vi "sub match keyword two value.vi"(8 "error in":errorcluster, 10 "keyword":string[](array[string]), 11 "string":string) -> (0 "error out":errorcluster, 2 "matched pairs (exist)":T1(array[cluster]), 3 "matched pairs (all)":T1(array[cluster]), 5 "remain string":string)   [LabVIEW 2018, in "Data Parser.lvclass"]
uses:
  Data Parser.lvclass
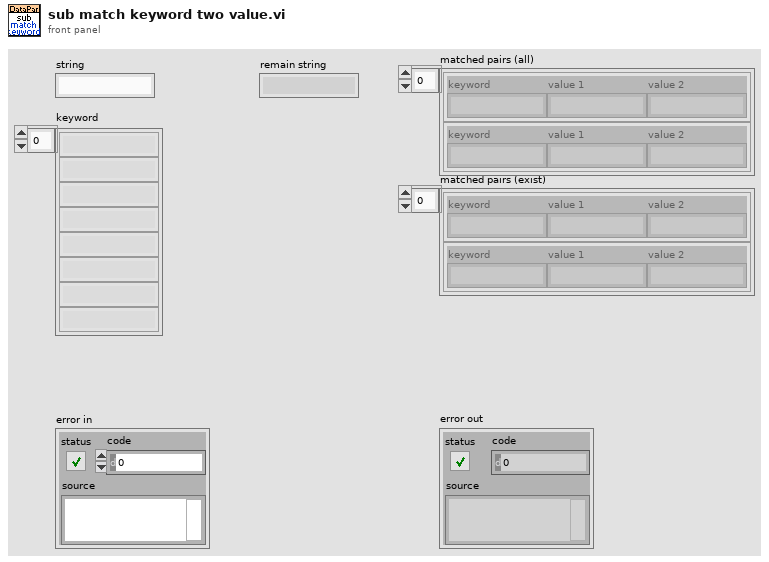
[diagram p1: front panel]
types:
  T1 = cluster{"keyword":string, "value 1":string, "value 2":string}[]
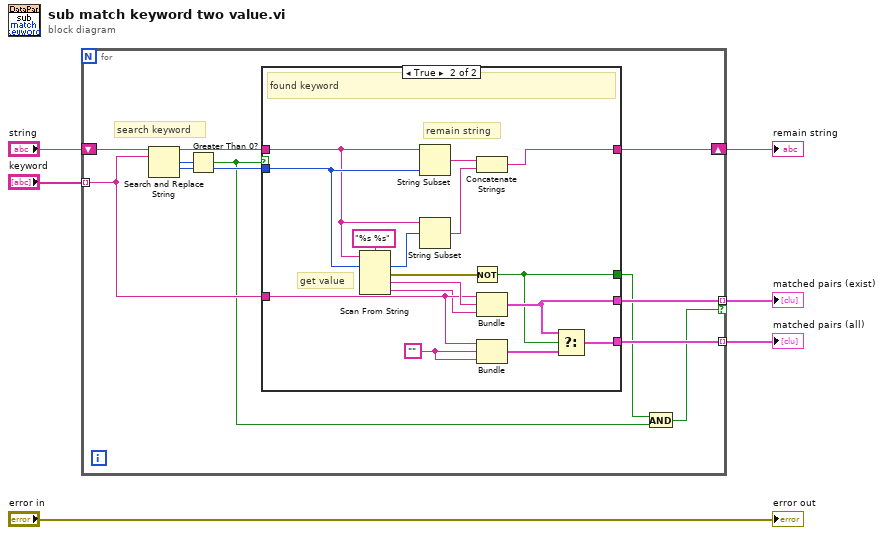
[diagram p0: block diagram]
diagram:
  n1 = for {
    tunnel: "keyword" -> [w12] mode=indexing
    shift-right: [w14] -> w3
    shift-left: "string" -> [w17]
    tunnel: [w13] -> w6 mode=indexing if=w7
    tunnel: [w11] -> w1 mode=indexing
    # "search keyword"
    n2 = Search and Replace String(input string=w17, search string=w12) -> (result string=w15:string, number of replacements=w10:i32, offset past replacement=w16:i32)  [unwired: 6 in, 1 out]
    n3 = Greater Than 0?(x=w10) -> (x > 0?=w9:bool)
    n4 = case shown="True" w9 {
      tunnel: w16 -> [_ w32]
      tunnel: w15 -> [w18 w31]
      tunnel: [w18 w27] -> w14
      tunnel: [_ w26] -> w13
      tunnel: w12 -> [_ w25]
      tunnel: [_ w23] -> w11
      tunnel: [_ w21] -> w8
      frame False {
        # "not found"
      }
      frame True {
        w20 = ""
        # "remain string"
        # "get value"
        # "found keyword"
        n5 = Scan From String(format string="%s %s", input string=w31, initial scan location=w32) -> (offset past scan=w30:u32, error out=w22:errorcluster, output 1=w33:string, output 2=w19:string)  [unwired: 3 in, 1 out]
        n6 = String Subset(string=w31, length (rest)=w32) -> (substring=w29:string)  [unwired: 1 in]
        n7 = String Subset(string=w31, offset (0)=w30) -> (substring=w28:string)  [unwired: 1 in]
        n8 = Not(x=w22) -> (.not. x?=w21:bool)
        n9 = Concatenate Strings(w29, w28) -> (w27:string)
        n10 = Bundle("String"=w25, w33, w19) -> (w26:cluster{"String":string, string, string})  [unwired: 1 in]
        n11 = Bundle("String"=w25, w20, w20) -> (w24:cluster{"String":string, string, string})  [unwired: 1 in]
        n12 = Select(t=w26, s=w21, f=w24) -> (s? t:f=w23:cluster{"String":string, string, string})
      }
    }
    n13 = And(x=w8, y=w9) -> (x .and. y?=w7:bool)
  }
  "matched pairs (exist)" <- w6
  "remain string" <- w3
  "matched pairs (all)" <- w1
  "error out" <- "error in"
